vi "TypeConv_Register Basic Types.vi"(11 "Type Categories":T1) -> (3 "Type Categories Dup":T1)   [LabVIEW 2013]
doc: "Copyright (c) 2016 Sze Howe Koh\n\nThis Source Code Form is subject to the terms of the Mozilla Public License, v. 2.0. If a copy of the MPL was not distributed with this file, You can obtain one at http://mozilla.org/MPL/2.0/."
uses:
  Data Structures/JSON/Type Categories.ctl
  Data Structures/JSON/TypeConv.ctl
  Data Structures/JSON/Simple Struct.ctl
  Data Structures/JSON/Param.ctl
  Data Structures/JSON/Method.ctl
  Data Structures/JSON/Connector Pane.ctl
  Data Structures/JSON/Connector Pane Terminal.ctl
  Data Structures/JSON/Class.ctl
  Data Structures/JSON/Enum.ctl
  Data Structures/JSON/Enum Value.ctl
  Data Structures/JSON/Property.ctl
  Action.ctl
  Category.ctl
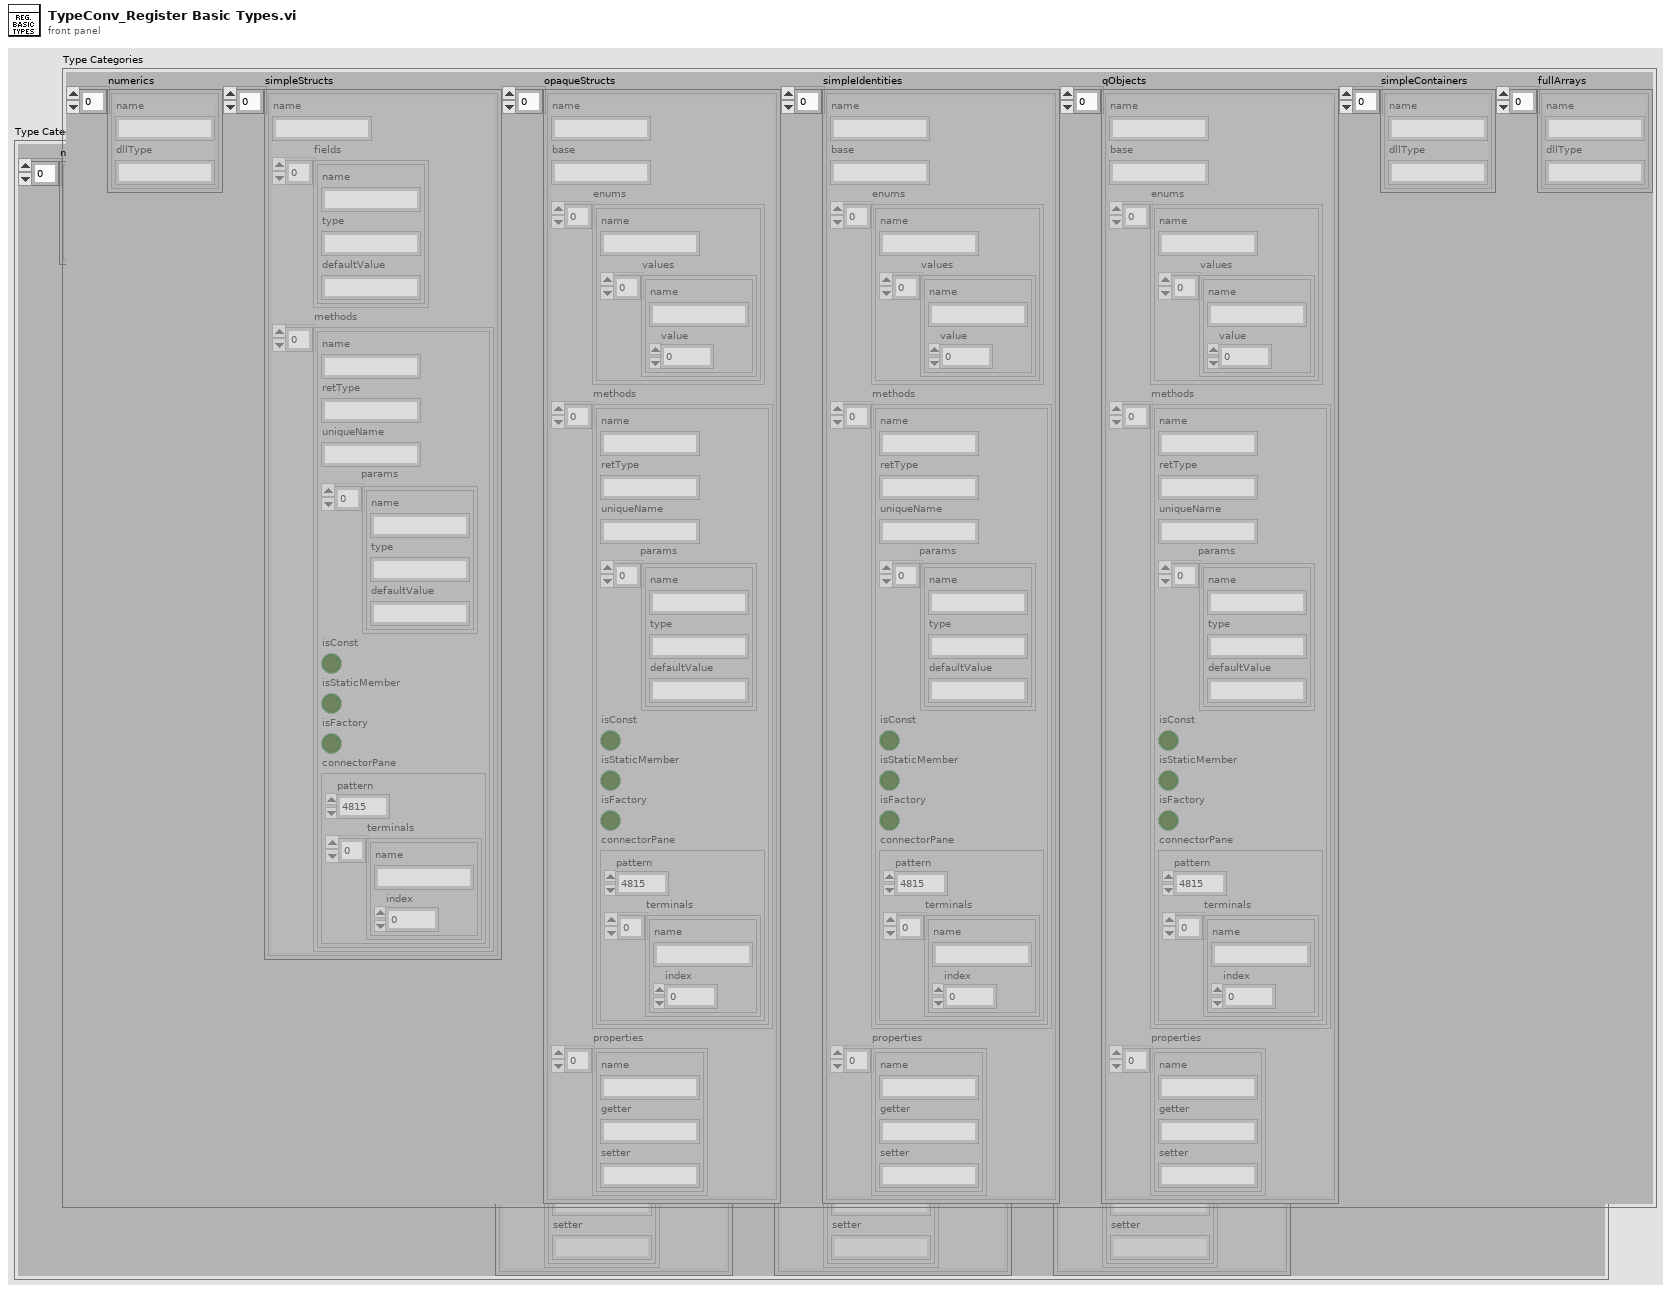
[diagram p1: front panel]
types:
  T1 = typedef "Type Categories.ctl" = cluster{"numerics":T2[], "simpleStructs":T3[], "opaqueStructs":T8[], "simpleIdentities":T8[], "qObjects":T8[], "simpleContainers":T2[], "fullArrays":T2[]}
  T2 = typedef "TypeConv.ctl" = cluster{"name":string, "dllType":string}
  T3 = typedef "Simple Struct.ctl" = cluster{"name":string, "fields":T4[], "methods":T5[]}
  T4 = typedef "Param.ctl" = cluster{"name":string, "type":string, "defaultValue":string}
  T5 = typedef "Method.ctl" = cluster{"name":string, "retType":string, "uniqueName":string, "params":T4[], "isConst":bool, "isStaticMember":bool, "isFactory":bool, "connectorPane":T6}
  T6 = typedef "Connector Pane.ctl" = cluster{"pattern":u32, "terminals":T7[]}
  T7 = typedef "Connector Pane Terminal.ctl" = cluster{"name":string, "index":u32}
  T8 = typedef "Class.ctl" = cluster{"name":string, "base":string, "enums":T9[], "methods":T5[], "properties":T11[]}
  T9 = typedef "Enum.ctl" = cluster{"name":string, "values":T10[]}
  T10 = typedef "Enum Value.ctl" = cluster{"name":string, "value":i32}
  T11 = typedef "Property.ctl" = cluster{"name":string, "getter":string, "setter":string}
  T12 = typedef "Category.ctl" = enum16{"Invalid", "Void", "Boolean", "Numeric", "Enum", "SimpleStruct", "OpaqueStruct", "SimpleIdentity", "QObject", "SimpleContainer", "FullArray"}
  T13 = typedef "Action.ctl" = enum16{"Register Type", "Register Projection", "Obtain Writer", "Get Projection", "Get Type Path", "Get Type Category"}
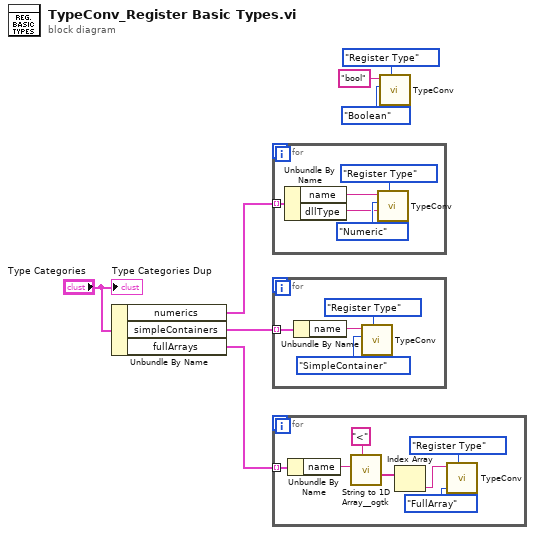
[diagram p0: block diagram]
diagram:
  n1 = Unbundle By Name("Type Categories") -> ("numerics"=w3:T2[], "simpleContainers"=w2:T2[], "fullArrays"=w1:T2[])
  n2 = for {
    tunnel: w3 -> [w12] mode=indexing
    n3 = Unbundle By Name(w12) -> ("name"=w11:string, "dllType"=w8:string)
    n4 = call "TypeConv.vi"("Action"=Action."Register Type", "Alternative Name"=w8, "Category"=Category."Numeric", "Type Name"=w11) -> ()  [unwired: 3 in, 5 out]
  }
  n5 = for {
    tunnel: w2 -> [w16] mode=indexing
    n6 = Unbundle By Name(w16) -> ("name"=w15:string)
    n7 = call "TypeConv.vi"("Action"=Action."Register Type", "Category"=Category."SimpleContainer", "Type Name"=w15) -> ()  [unwired: 4 in, 5 out]
  }
  n8 = for {
    tunnel: w1 -> [w23] mode=indexing
    n9 = Unbundle By Name(w23) -> ("name"=w18:string)
    n10 = call <userlib>:"String to 1D Array__ogtk.vi"("delimiter (Tab)"="<", "string"=w18) -> ("Array of Strings"=w19:string[])  [unwired: 9 in]
    n11 = Index Array(array=w19) -> (element=w17:string)  [unwired: 1 in]
    n12 = call "TypeConv.vi"("Action"=Action."Register Type", "Category"=Category."FullArray", "Type Name"=w17) -> ()  [unwired: 4 in, 5 out]
  }
  n13 = call "TypeConv.vi"("Action"=Action."Register Type", "Category"=Category."Boolean", "Type Name"="bool") -> ()  [unwired: 4 in, 5 out]
  "Type Categories Dup" <- "Type Categories"
